vi "Areotech set positon.vi"(8 "error in (no error)":errorcluster, 10 "Parsed CMD":T1, 11 "AerotechStage in":refnum<class "AerotechStage.lvclass">) -> (0 "error out":errorcluster, 2 "new commands":string, 3 "AerotechStage out":refnum<class "AerotechStage.lvclass">)   [LabVIEW 2020, in "AerotechStage.lvclass"]
uses:
  AerotechStage.lvclass
  parsed device cmd.ctl
  AerotechStage.lvclass/AerotechStage.ctl
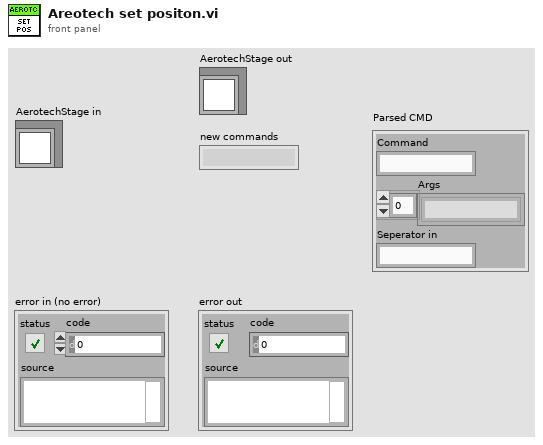
[diagram p1: front panel]
types:
  T1 = typedef "parsed device cmd.ctl" = cluster{"Command":string, "Args":string[], "Seperator in":string}
  T2 = typedef "OnOffTypeDef.ctl" = enum16{"off", "on"}
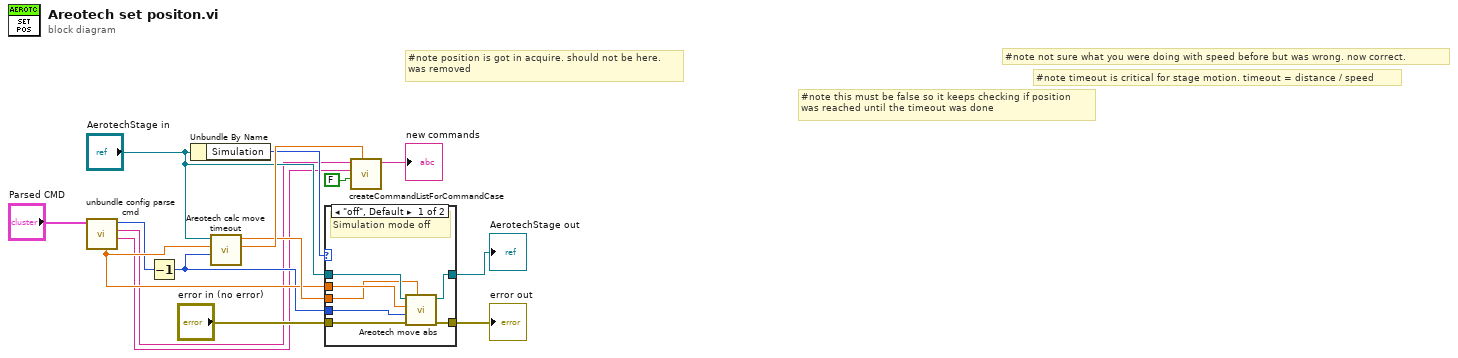
[diagram p0: block diagram]
diagram:
  # "#note timeout is critical for stage motion. timeout = distance / speed"
  # "#note not sure what you were doing with speed before but was wrong. now correct."
  # "#note this must be false so it keeps checking if position\nwas reached until the timeout was done"
  # "#note position is got in acquire. should not be here.\nwas removed"
  n1 = call "unbundle config parse cmd.vi"("Parsed CMD"="Parsed CMD") -> ("Value string"=w5:string, "Command"=w3:string, "Channel number not index"=w7:i32, "Value double"=w13:dbl)  [unwired: 7 in]
  n2 = Decrement(x=w7) -> (x-1=w12:i32)
  n3 = Unbundle By Name("AerotechStage in") -> ("Simulation"=w6:T2)
  n4 = call "Areotech calc move timeout.vi"("Numeric in"=w12, "Position"=w13, "AerotechStage in"="AerotechStage in") -> ("Numeric out"=w15:dbl, "Value"=w14:dbl)  [unwired: 7 in]
  n5 = case shown="\"off\", Default" w6 {
    tunnel: w13 -> [w21 _]
    tunnel: "AerotechStage in" -> [w22 w23]
    tunnel: "error in (no error)" -> [w19 w24]
    tunnel: [w20 w24] -> w9
    tunnel: [w17 w23] -> w10
    tunnel: w12 -> [w16 _]
    tunnel: w14 -> [w18 _]
    frame "off", Default {
      # "Simulation mode off"
      n6 = call "Areotech move abs.vi"("speed"=w18, "error in (no error)"=w19, "stage index"=w16, "position"=w21, "AerotechStage in"=w22) -> ("error out"=w20:errorcluster, "AerotechStage out"=w17:refnum<class "AerotechStage.lvclass">)  [unwired: 5 in]
    }
    frame "on" {
      # "Simulation mode on"
    }
  }
  "AerotechStage out" <- w10
  "error out" <- w9
  n7 = call "createCommandListForCommandCase.vi"("timeout (optional)"=w15, "immediate Check (only once)"=FALSE, "setvalue"=w5, "command"=w3) -> ("new commands"=→"new commands":string)  [unwired: 7 in]
